vi "Destructor.vi"(8 "error in (no error)":errorcluster, 11 "Agilent 3458A in":refnum<class "Agilent 3458A.lvclass">) -> (0 "error out":errorcluster, 3 "Agilent 3458A out":refnum<class "Agilent 3458A.lvclass">)   [LabVIEW 2011, in "Agilent 3458A.lvclass"]
uses:
  Agilent 3458A.lvclass
  <instrlib>/Agilent 3458/Agilent 3458.lvlib
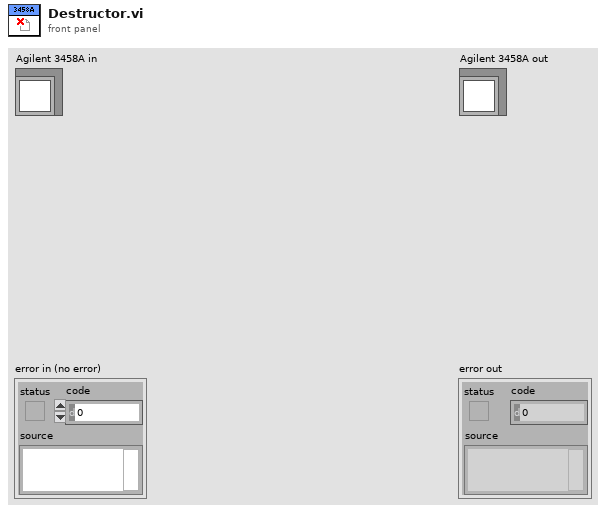
[diagram p1: front panel]
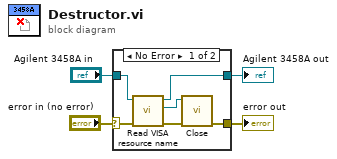
[diagram p0: block diagram]
diagram:
  n1 = case shown="No Error" "error in (no error)" {
    selector: "error in (no error)" -> [w7 w12]
    tunnel: [w8 w12] -> w3
    tunnel: [w5 w11] -> w1
    tunnel: "Agilent 3458A in" -> [w9 w11]
    frame No Error {
      n2 = call-dynamic "Read VISA resource name.vi"("error in (no error)"=w7, "Multimeter in"=w9) -> ("error out"=w6:errorcluster, "VISA resource name"=w10:refnum<visa-resource-name>, "Multimeter out"=w5:refnum<class "Agilent 3458A.lvclass">)  [unwired: 7 in]
      n3 = call <instrlib>:"Close.vi"("error in (no error)"=w6, "VISA resource name"=w10) -> ("error out"=w8:errorcluster)  [unwired: 9 in]
    }
    frame Error {
    }
  }
  "error out" <- w3
  "Agilent 3458A out" <- w1
